vi "ep_Check Signaling Settings.vi"(8 "error in (no error)":errorcluster, 11 "signaling voltage event settings":T1={"detection threshold [%]"=0.3, "start logical 1 length [s]"=2.99, "start logical 0 length [s]"=2.33, "maximum event length [s]"=64.0}) -> (0 "error out":errorcluster)   [LabVIEW 2014, in "NI_EP_Power Quality.lvlib"]
uses:
  <vilib>/addons/Electrical Power/PQ/NI_EP_Power Quality.lvlib
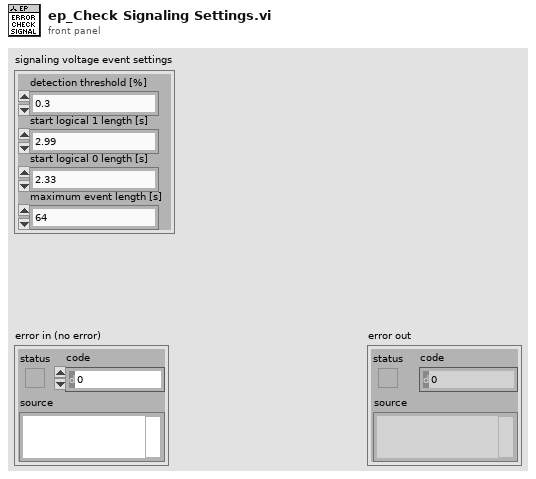
[diagram p1: front panel]
types:
  T1 = cluster{"detection threshold [%]":dbl, "start logical 1 length [s]":dbl, "start logical 0 length [s]":dbl, "maximum event length [s]":dbl}
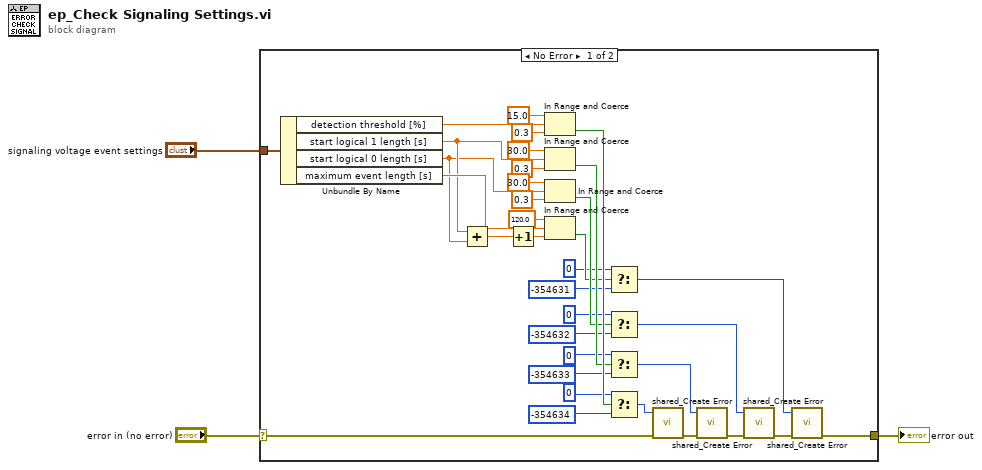
[diagram p0: block diagram]
diagram:
  n1 = case shown="No Error" "error in (no error)" {
    selector: "error in (no error)" -> [w5 w39]
    tunnel: "signaling voltage event settings" -> [w27 _]
    tunnel: [w4 w39] -> w1
    frame No Error {
      n2 = Unbundle By Name(w27) -> ("detection threshold [%]"=w35:dbl, "start logical 1 length [s]"=w24:dbl, "start logical 0 length [s]"=w23:dbl, "maximum event length [s]"=w29:dbl)
      n3 = Add(x=w24, y=w23) -> (x+y=w22:dbl)
      n4 = Increment(x=w22) -> (x+1=w21:dbl)
      n5 = In Range and Coerce(upper limit=15.0, x=w35, lower limit=0.3) -> (In Range?=w38:bool)  [unwired: 1 out]
      n6 = In Range and Coerce(upper limit=30.0, x=w24, lower limit=0.3) -> (In Range?=w32:bool)  [unwired: 1 out]
      n7 = In Range and Coerce(upper limit=30.0, x=w23, lower limit=0.3) -> (In Range?=w31:bool)  [unwired: 1 out]
      n8 = In Range and Coerce(upper limit=120.0, x=w29, lower limit=w21) -> (In Range?=w28:bool)  [unwired: 1 out]
      n9 = Select(t=0 ("error code (0)"), s=w28, f=-354631 ("error code (0)")) -> (s? t:f=w6:i32)
      n10 = Select(t=0 ("error code (0)"), s=w31, f=-354632 ("error code (0)")) -> (s? t:f=w9:i32)
      n11 = Select(t=0 ("error code (0)"), s=w32, f=-354633 ("error code (0)")) -> (s? t:f=w12:i32)
      n12 = Select(t=0 ("error code (0)"), s=w38, f=-354634 ("error code (0)")) -> (s? t:f=w15:i32)
      n13 = call <vilib>:"shared_Create Error.vi"("error in (no error)"=w5, "error code (0)"=w15) -> ("error out"=w13:errorcluster)  [unwired: 9 in]
      n14 = call <vilib>:"shared_Create Error.vi"("error in (no error)"=w13, "error code (0)"=w12) -> ("error out"=w10:errorcluster)  [unwired: 9 in]
      n15 = call <vilib>:"shared_Create Error.vi"("error in (no error)"=w10, "error code (0)"=w9) -> ("error out"=w7:errorcluster)  [unwired: 9 in]
      n16 = call <vilib>:"shared_Create Error.vi"("error in (no error)"=w7, "error code (0)"=w6) -> ("error out"=w4:errorcluster)  [unwired: 9 in]
    }
    frame Error {
    }
  }
  "error out" <- w1
